vi "Edgertronic-:get_camstatus copy.vi"(5 "Setup":T2={"URL"="130.64.16.195", "remote port"=80, "mode (standard)"=enum."Standard"}) -> (0 "error out":errorcluster, 1 "Cam Status:":T1={"Level"="20140911165611", "Flags"="20140911165611", "Is Temp"="20140911165611", "FPGA Temp"="20140911165611", "State"="20140911165611", "Camera Time"="20140911165611", "dacvrefadc"="20140911165611", "Connection Information:"=""}, 2 "data out":string="HTTP/1.0 200 OK\r\nContent-Type: text/html; charset=utf-8\r\nContent-Length: 313\r\nConnection: close\r\nDate: Tue, 16 Jun 2015 13:54:12 GMT\r\nServer: lighttpd/1.4.11 (edgertonic slow motion camera)\r\n\r\n{\"build_date\": \"20150112\", \"sw_build_date\": \"20140911165611\", \"fpga_initialized\": 1, \"hardware_revision\": 6, \"model_number\": 1, \"home_dir\": \"/home/root/ss-web\", \"ir_filter\": 1, \"mac_addr\": \"00:1B:C5:09:61:4D\", \"serial_console_enabled\": false, \"serial_number\": 333, \"fpga_version\": 70, \"hardware_configuration\": 1}")   [LabVIEW 2012]
doc: "This VI returns the camera status information."
panel:
  in  "GET Cmd":string="/get_camstatus"
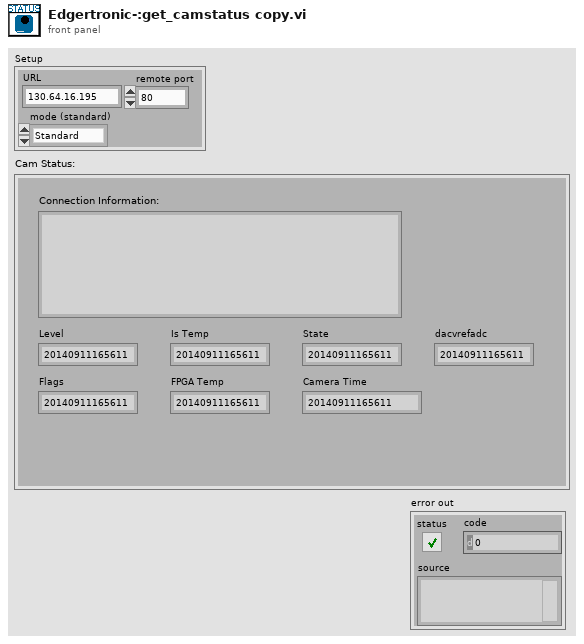
[diagram p1: front panel]
types:
  T1 = cluster{"Level":string, "Flags":string, "Is Temp":string, "FPGA Temp":string, "State":string, "Camera Time":string, "dacvrefadc":string, "Connection Information:":string}
  T2 = cluster{"URL":string, "remote port":u16, "mode (standard)":enum16{"Standard", "Buffered", "CRLF", "Immediate"}}
  T3 = cluster{"Parameter":string, "Parameter 2":string, "Parameter 3":string, "Parameter 4":string, "Parameter 5":string, "Parameter 6":string, "Parameter 7":string, string, string, string, string, string, string, string, string, string, string, string, string, string, string, string, string, string, string, string, string, string, string, string, string, string, string, string, string, string}
  T4 = cluster{"[0]":string, "[1]":string, "[2]":string, "[3]":string, "[4]":string, "[5]":string, "[6]":string, "[7]":string, "[8]":string, "[9]":string, "[10]":string, "[11]":string, "[12]":string, "[13]":string, "[14]":string, "[15]":string, "[16]":string, "[17]":string, "[18]":string, "[19]":string, "[20]":string, "[21]":string, "[22]":string, "[23]":string, "[24]":string, "[25]":string, "[26]":string, "[27]":string, "[28]":string, "[29]":string, "[30]":string, "[31]":string, "[32]":string, "[33]":string, "[34]":string, "[35]":string}
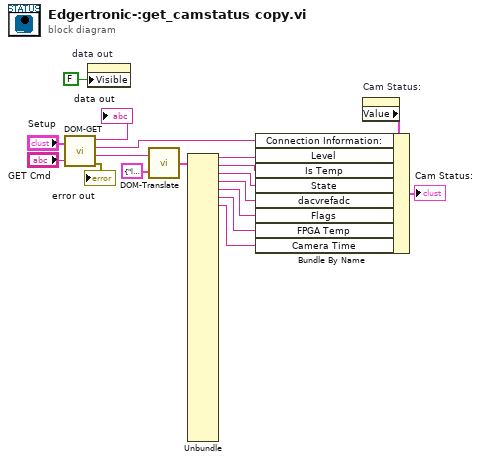
[diagram p0: block diagram]
diagram:
  n1 = call <userlib>:"DOM-GET.vi"("Setup"="Setup", "GET Command"="GET Cmd") -> ("Data Out from Camera"=→"data out":string, "Connection Information"=w12:string, "Value String"=w10:string, "error out"=→"error out":errorcluster)
  n2 = property on="data out" class="Str"("Visible"=FALSE) -> ()  [unwired: 2 in, 2 out]
  n3 = call <userlib>:"DOM-Translate.vi"("Parameter Cluster in"=T3 {"Parameter"="level", "Parameter 2"="is_temp", "Parameter 3"="state", "Parameter 4"="dacvrefadc", "Parameter 5"="flags", "Parameter 6"="fpga_temp", "Parameter 7"="camera_time", "", "", "", "", "", "", "", "", "", "", "", "", "", "", "", "", "", "", "", "", "", "", "", "", "", "", "", "", ""}, "Value Data in"=w10) -> ("Value Cluster out"=w8:T4)
  n4 = Unbundle(w8) -> ("[0]"=w7:string, "[1]"=w6:string, "[2]"=w5:string, "[3]"=w4:string, "[4]"=w3:string, "[5]"=w2:string, "[6]"=w1:string)  [unwired: 29 out]
  n5 = property on="Cam Status:" class="Clust (strict)"() -> ("Value"=w9:T1)  [unwired: 2 in, 2 out]
  n6 = Bundle By Name(cluster=w9, "Connection Information:"=w12, "Level"=w7, "Is Temp"=w6, "State"=w5, "dacvrefadc"=w4, "Flags"=w3, "FPGA Temp"=w2, "Camera Time"=w1) -> (→"Cam Status:":T1)
